vi "矩阵乘法.vi"() -> ()   [LabVIEW 2018]
uses:
  <vilib>/Analysis/Matrix/Datatypes/RealMatrix.ctl
  <vilib>/Analysis/baseanly.llb/Real A x B.vi
  <vilib>/Analysis/NI_AALBase.lvlib
  <vilib>/Analysis/Matrix/NI_Matrix.lvlib
panel:
  out "A x B":T1 caption="矩阵A x B"
  in  "Real Matrix 2":T1 caption="实数矩阵"
  in  "Real Matrix":T1 caption="实数矩阵"
  out "字符串":string="矩阵的乘法是两个矩阵或一个矩阵与输入向量相乘。"
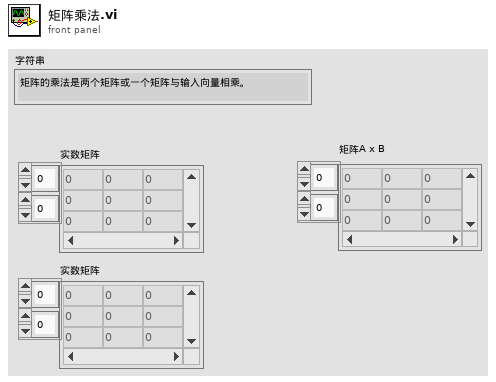
[diagram p1: front panel]
types:
  T1 = typedef "NI_Matrix.lvlib/RealMatrix.ctl" = dbl[][]
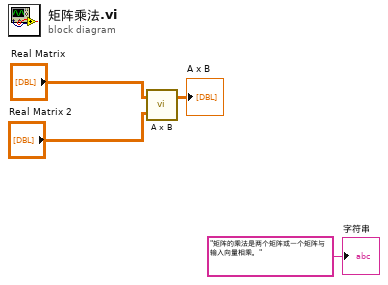
[diagram p0: block diagram]
diagram:
  n1 = call-poly <vilib>:"A x B.vi"("B"="Real Matrix 2", "A"="Real Matrix") -> ("A x B"=→"A x B":T1)  [unwired: 1 out]
  "字符串" <- "矩阵的乘法是两个矩阵或一个矩阵与输入向量相乘。"
